vi "ClsterIO.vi"() -> ()   [LabVIEW 2020]
panel:
  out "data":T1
  in  "Cluster":T1
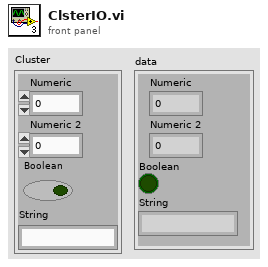
[diagram p1: front panel]
types:
  T1 = cluster{"Numeric":dbl, "Numeric 2":dbl, "Boolean":bool, "String":string}
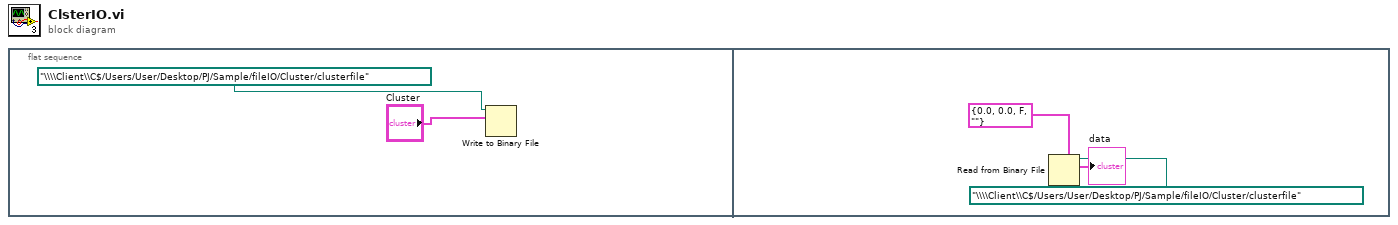
[diagram p0: block diagram]
diagram:
  n1 = flat-sequence {
    frame #0 {
      n2 = Write to Binary File(file (use dialog)=path "\\\\Client\\C$/Users/User/Desktop/PJ/Sample/fileIO/Cluster/clusterfile" ("file path (dialog if empty)"), data="Cluster") -> ()  [unwired: 4 in, 3 out]
    }
    frame #1 {
      n3 = Read from Binary File(5:T1 {"Numeric"=0.0, "Numeric 2"=0.0, "Boolean"=FALSE, "String"=""} ("Cluster"), 11:path "\\\\Client\\C$/Users/User/Desktop/PJ/Sample/fileIO/Cluster/clusterfile" ("file path (dialog if empty)")) -> (2:→"data":T1)  [unwired: 4 in, 3 out]
    }
  }
